vi "Extract Timestamp from RxUDP Header.vi"(11 "header in":u32[](array[numeric])) -> (0 "IrigTime out":T1, 1 "time stamp out":timestamp, 2 "seconds out":dbl, 3 "header out":u32[](array[numeric]))   [LabVIEW 2020]
uses:
  Program Files/National Instruments/LabVIEW 2025/instr.lib/AIM GmbH/_AIM 664/AIM664LV.lvlib
  Program Files/National Instruments/LabVIEW 2025/instr.lib/AIM GmbH/_AIM 664/bsp/Controls/IrigTime.ctl
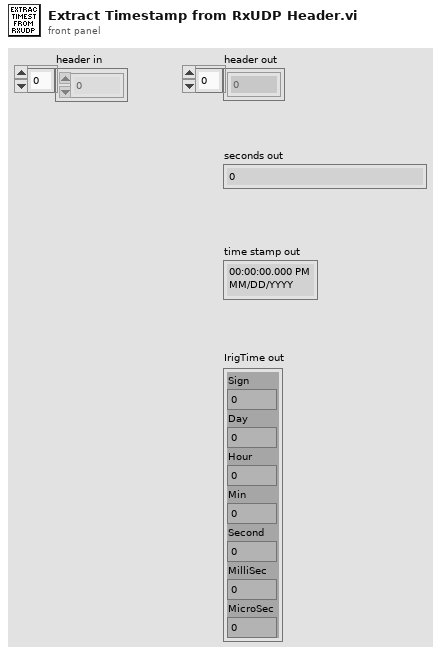
[diagram p1: front panel]
types:
  T1 = typedef "AIM664LV.lvlib/IrigTime.ctl" = cluster{"Sign":i32, "Day":u32, "Hour":u32, "Min":u32, "Second":u32, "MilliSec":u32, "MicroSec":u32}
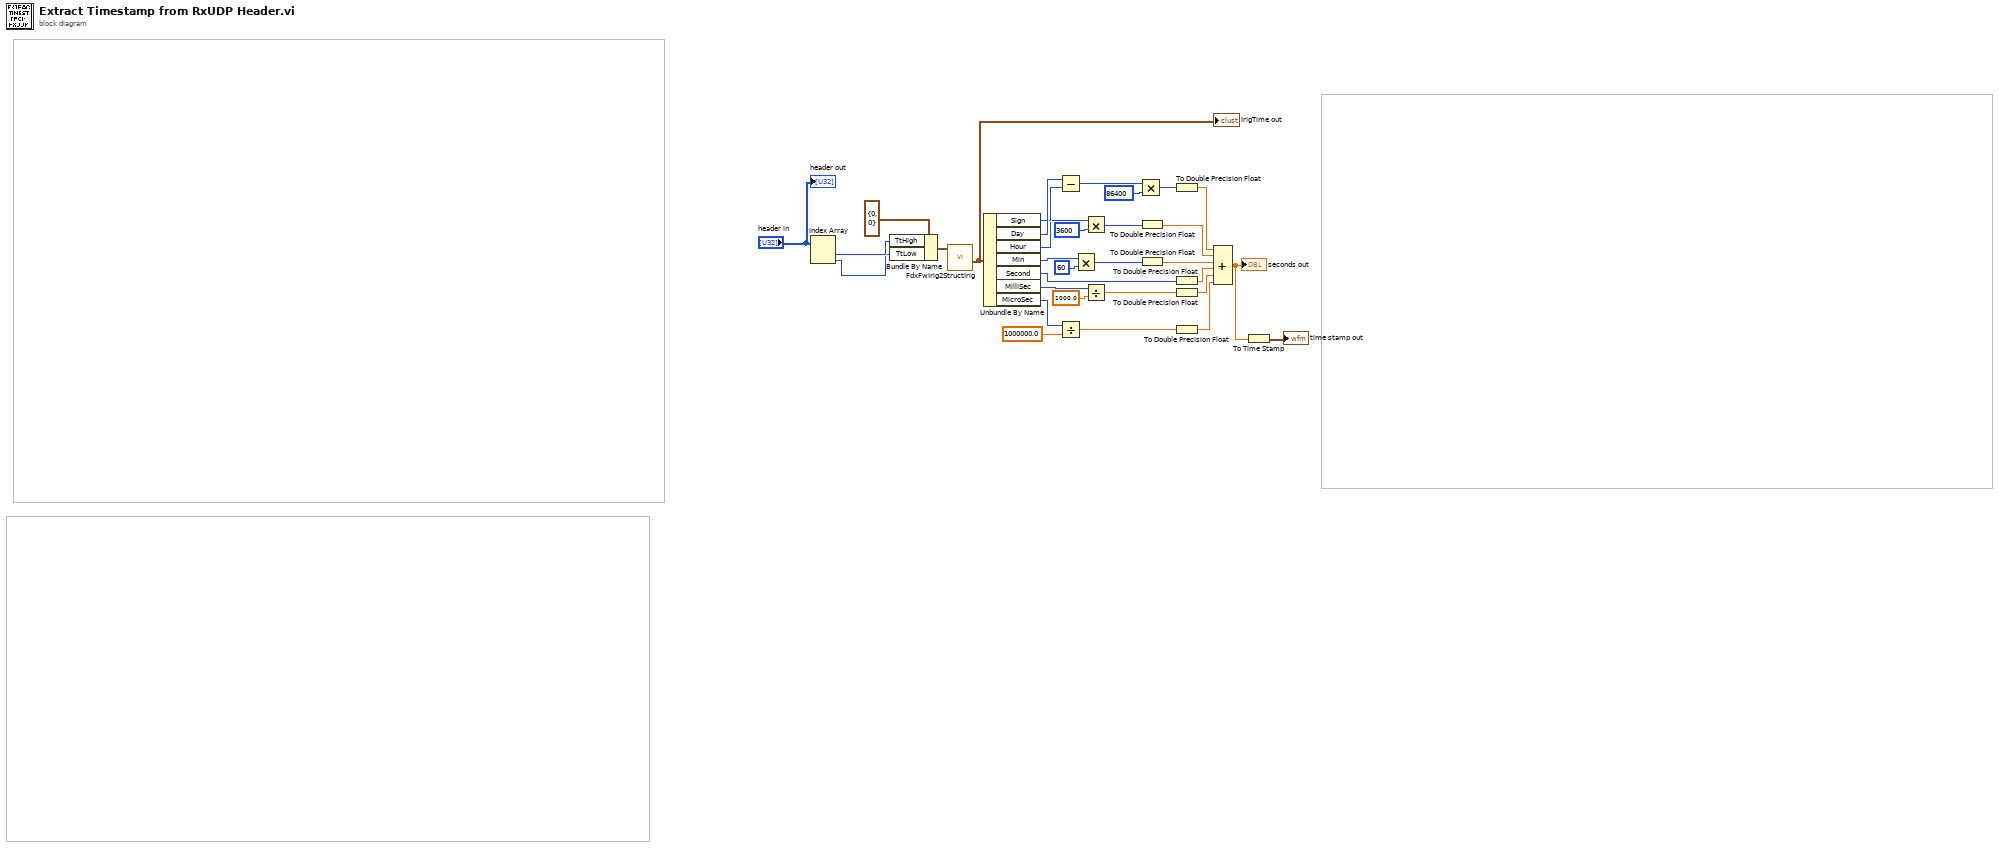
[diagram p0: block diagram]
diagram:
  n1 = Index Array(array="header in") -> (element #1=w29:u32, element #2=w28:u32)  [unwired: 2 in]
  n2 = Bundle By Name(cluster=cluster{"TtHigh":u32, "TtLow":u32} {"TtHigh"=0, "TtLow"=0} ("FwIrigTime"), "TtHigh"=w29, "TtLow"=w28) -> (w30:cluster{"TtHigh":u32, "TtLow":u32})
  n3 = call "FdxFwIrig2StructIrig.vi"("FwIrigTime"=w30) -> ("IrigTime"=w27:T1)  [unwired: 9 in, 1 out]
  "IrigTime out" <- w27
  n4 = Unbundle By Name(w27) -> ("Sign"=w25:i32, "Day"=w26:u32, "Hour"=w22:u32, "Min"=w21:u32, "Second"=w13:u32, "MilliSec"=w7:u32, "MicroSec"=w9:u32)
  n5 = Subtract(x=w26, y=w25) -> (x-y=w24:u32)
  n6 = Divide(x=w9, y=1000000.0) -> (x/y=w5:dbl)
  n7 = Multiply(x=w21, y=u32 60) -> (x*y=w14:u32)
  n8 = Multiply(x=w22, y=u32 3600) -> (x*y=w18:u32)
  n9 = Divide(x=w7, y=1000.0) -> (x/y=w6:dbl)
  n10 = Multiply(x=w24, y=u32 86400) -> (x*y=w19:u32)
  n11 = To Double Precision Float(number=w18) -> (double precision float=w16:dbl)
  n12 = To Double Precision Float(number=w14) -> (double precision float=w15:dbl)
  n13 = To Double Precision Float(number=w19) -> (double precision float=w17:dbl)
  n14 = To Double Precision Float(number=w13) -> (double precision float=w12:dbl)
  n15 = To Double Precision Float(number=w6) -> (double precision float=w4:dbl)
  n16 = To Double Precision Float(number=w5) -> (double precision float=w3:dbl)
  n17 = Compound Arithmetic op=ADD(w17, w16, w15, w12, w4, w3) -> (w2:dbl)
  "seconds out" <- w2
  n18 = To Time Stamp(1:w2) -> (0:→"time stamp out":timestamp)
  "header out" <- "header in"
